vi "Start Scorer.vi"(8 "error in (no error)":errorcluster, 9 "Submission":refnum<class "Submission.lvclass">, 10 "Scorer In":refnum<class "Scorer.lvclass">, 11 "SOL-Server in":refnum<class "SOL-Server.lvclass">) -> (0 "error out":errorcluster, 2 "Scorer":refnum<class "Scorer.lvclass">, 3 "SOL-Server out":refnum<class "SOL-Server.lvclass">)   [LabVIEW 2020, in "Summer of LabVIEW.lvlib" / "SOL-Server.lvclass"]
uses:
  SOL-Server.lvclass
  Scorer/Scorer.lvclass
  Submission/Submission.lvclass
  SOL-Server.lvclass/SOL-Server.ctl
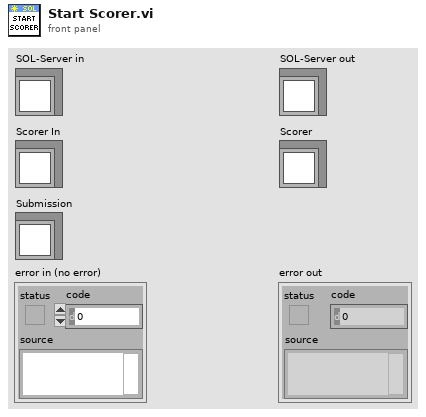
[diagram p1: front panel]
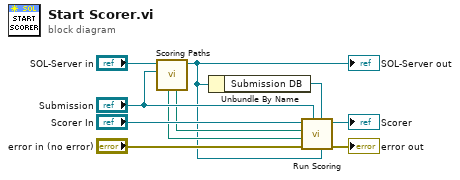
[diagram p0: block diagram]
diagram:
  n1 = call "Scoring Paths.vi"("Submission"="Submission", "SOL-Server in"="SOL-Server in") -> ("SOL-Server out"=w2:refnum<class "SOL-Server.lvclass">, "LLB Path"=w4:path, "Scorer Path"=w3:path)  [unwired: 6 in, 1 out]
  "SOL-Server out" <- w2
  n2 = Unbundle By Name(w2) -> ("Submission DB"=w1:refnum<class "Submission DB.lvclass">)
  n3 = call "Run Scoring.vi"("Server"=w2, "Submission DB"=w1, "Submission"="Submission", "error in (no error)"="error in (no error)", "Scorer Path"=w3, "LLB Path"=w4, "Scorer in"="Scorer In") -> ("error out"=→"error out":errorcluster, "Scorer out"=→"Scorer":refnum<class "Scorer.lvclass">)  [unwired: 3 in]
